vi "EMV First Last Difference.vi"(8 "error in (no error)":errorcluster, 11 "Current T6 Temperatures in":dbl[](array[numeric])) -> (0 "error out":errorcluster, 1 "First - Row 8":dbl, 2 "First - Row 9":dbl, 3 "First - Row 10":dbl, 5 "Current Temperature":dbl)   [LabVIEW 2016]
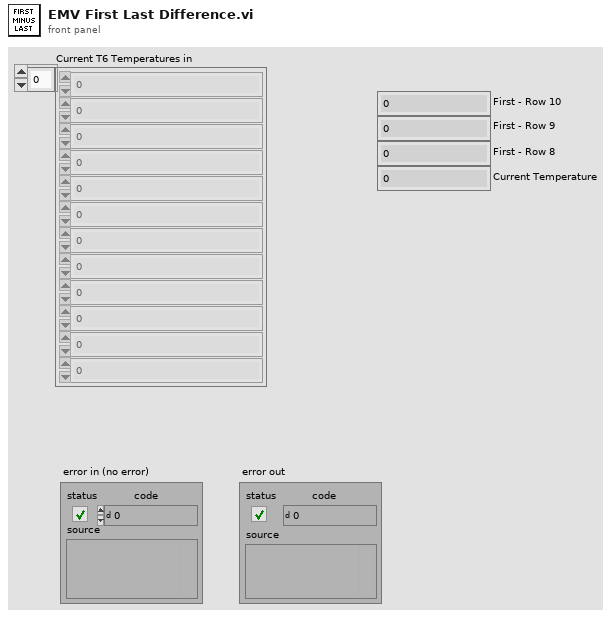
[diagram p1: front panel]
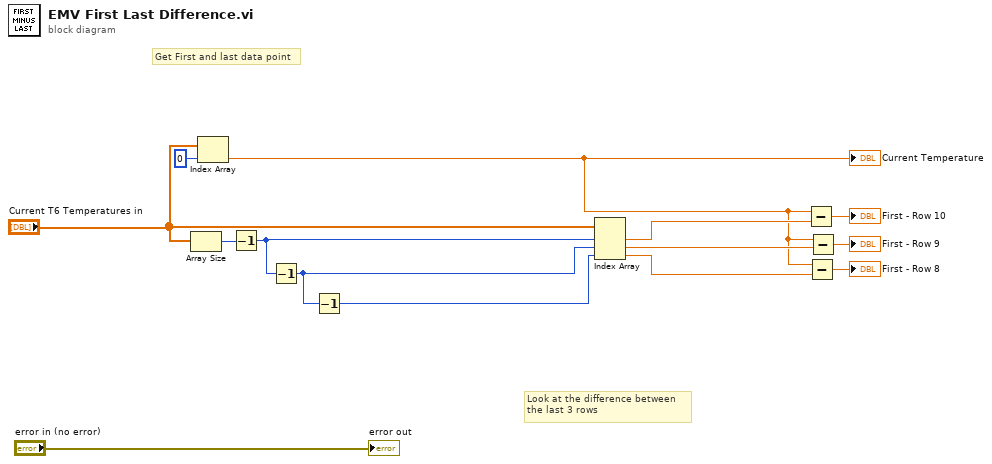
[diagram p0: block diagram]
diagram:
  # "Look at the difference between\nthe last 3 rows"
  # "Get First and last data point"
  n1 = Array Size(array="Current T6 Temperatures in") -> (size(s)=w12:i32)
  n2 = Index Array(array="Current T6 Temperatures in", index=0) -> (element=w4:dbl)
  "Current Temperature" <- w4
  n3 = Decrement(x=w12) -> (x-1=w9:i32)
  n4 = Decrement(x=w9) -> (x-1=w7:i32)
  n5 = Decrement(x=w7) -> (x-1=w8:i32)
  n6 = Index Array(array="Current T6 Temperatures in", index #1=w9, index #2=w7, index #3=w8) -> (element #1=w14:dbl, element #2=w5:dbl, element #3=w3:dbl)
  n7 = Subtract(x=w4, y=w14) -> (x-y=→"First - Row 10":dbl)
  n8 = Subtract(x=w4, y=w3) -> (x-y=→"First - Row 8":dbl)
  n9 = Subtract(x=w4, y=w5) -> (x-y=→"First - Row 9":dbl)
  "error out" <- "error in (no error)"
